vi "Pad Array.vi"(7 "default element":dbl format="%#_13g", 9 "Pulse delay":i32, 10 "Desired size":i32=8192, 11 "Signal in":dbl[](array[numeric])) -> (3 "Signal out":dbl[](array[numeric]))   [LabVIEW 2025]
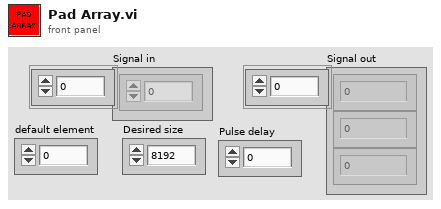
[diagram p1: front panel]
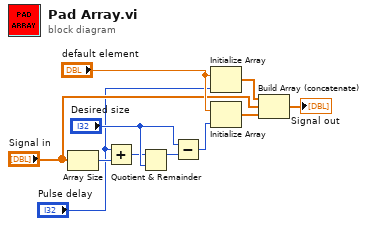
[diagram p0: block diagram]
diagram:
  n1 = Array Size(array="Signal in") -> (size(s)=w6:i32)
  n2 = Add(x="Pulse delay", y=w6) -> (x+y=w2:i32)
  n3 = Quotient & Remainder(x=w2, y="Desired size") -> (x-y*floor(x/y)=w8:i32)  [unwired: 1 out]
  n4 = Subtract(x="Desired size", y=w8) -> (x-y=w10:i32)
  n5 = Initialize Array("default element", "Pulse delay") -> (w3:dbl[])
  n6 = Initialize Array("default element", w10) -> (w9:dbl[])
  n7 = Build Array (concatenate)(w3, "Signal in", w9) -> (→"Signal out":dbl[])
